vi "Read Dispatcher Response.vi"(8 "error in (no error)":errorcluster, 9 "timeout in ms (0)":i32 format="%d ms", 11 "Dispatcher Interface in":refnum<class "Dispatcher Interface.lvclass">) -> (0 "error out":errorcluster, 2 "response":T1, 3 "Dispatcher Interface out":refnum<class "Dispatcher Interface.lvclass">, 4 "# elements":u32)   [LabVIEW 2017, in "DSF Core.lvlib" / "Dispatcher Interface.lvclass"]
uses:
  Dispatcher Interface.lvclass
  C:/Users/Admin/Desktop/Data Sharing Framework/Source/Core/Engine/Classes/Interfaces/Interface/Interface.lvclass
  Response Data.ctl
  Response.ctl
  Parameters.ctl
  Interface/Interface.lvclass/Interface.ctl
  Interface/Read RT FIFO.vi
  Response Timeout.vi
  Interface/Interface.lvclass
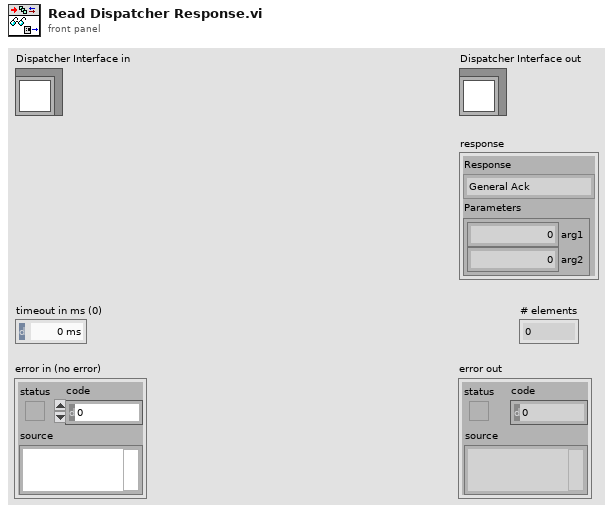
[diagram p1: front panel]
types:
  T1 = typedef "DSF Core.lvlib/Dispatcher Interface.lvclass/Response Data.ctl" = cluster{"Response":T2, "Parameters":T3}
  T2 = typedef "DSF Core.lvlib/Dispatcher Interface.lvclass/Response.ctl" = enum8{"General Ack", "Error", "Shutting Down"}
  T3 = typedef "DSF Core.lvlib/Dispatcher Interface.lvclass/Parameters.ctl" = cluster{"arg1":u64, "arg2":u64}
  T4 = typedef "DSF Core.lvlib/Interface.lvclass/RT FIFO Data.ctl" = cluster{"Command":u8, "Payload":T5}
  T5 = typedef "DSF Core.lvlib/Interface.lvclass/RT FIFO Parameters.ctl" = cluster{"arg1":u64, "arg2":u64}
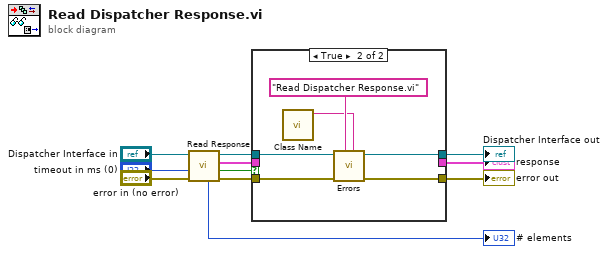
[diagram p0: block diagram]
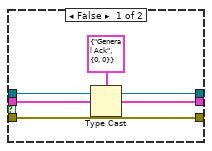
[diagram p2: hidden frame]
diagram:
  n1 = call "Read Response.vi"("error in (no error)"="error in (no error)", "timeout in ms (0)"="timeout in ms (0)", "Interface in"="Dispatcher Interface in") -> ("error out"=w6:errorcluster, "timed out?"=w5:bool, "response"=w2:T4, "Interface out"=w7:refnum<class "Dispatcher Interface.lvclass">, "# elements"=→"# elements":u32)  [unwired: 4 in]
  n2 = case shown="True" w5 {
    tunnel: w6 -> [w15 w21]
    tunnel: w7 -> [w16 w18]
    tunnel: [w16 w20] -> w4
    tunnel: [w15 w19] -> w3
    tunnel: w2 -> [w12 _]
    tunnel: [w13 _] -> w1
    frame False {
      n3 = Type Cast(type=T1 {"Response"=enum."General Ack", "Parameters"={"arg1"=0, "arg2"=0}} ("Dispatcher Response"), x=w12) -> (*(type *) &x=w13:T1)
    }
    frame True {
      n4 = call "Class Name.vi"() -> ("class name"=w17:string)  [unwired: 11 in]
      n5 = call-poly "Errors.vi"("error source class name"=w17, "error source vi name"="Read Dispatcher Response.vi", "error in (no error)"=w21, "Interface in"=w18) -> ("error out"=w19:errorcluster, "Interface out"=w20:refnum<class "Dispatcher Interface.lvclass">)  [unwired: 6 in]
    }
  }
  "error out" <- w3
  "Dispatcher Interface out" <- w4
  "response" <- w1
